vi "CaseStructures.vi"() -> ()   [LabVIEW 2021]
panel:
  in  "Enum":enum16{"Add", "Subtract", "Multiply", "Divide"}(ring)
  in  "stop":bool
  out "Answer":dbl
  in  "Numeber 2":dbl
  in  "Number 1":dbl
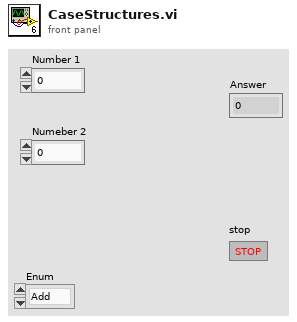
[diagram p1: front panel]
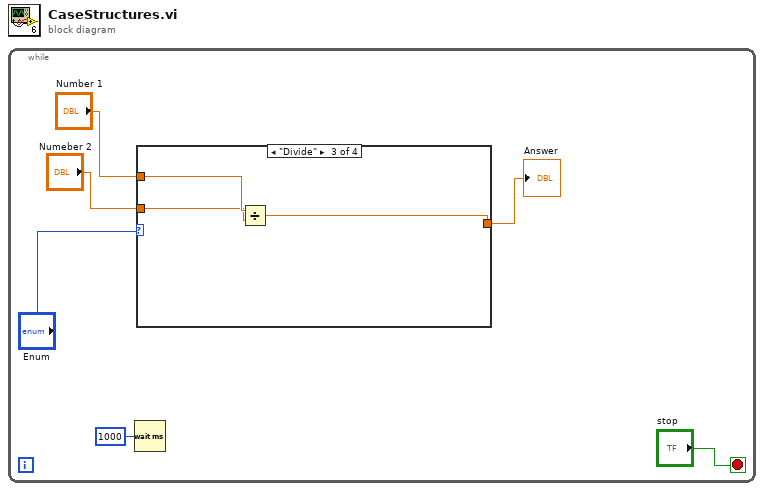
[diagram p0: block diagram]
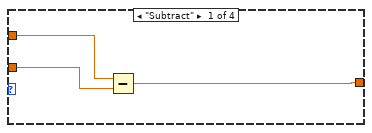
[diagram p2: hidden frame]
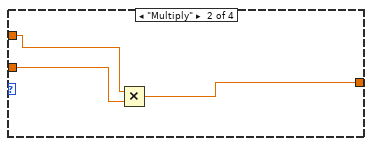
[diagram p3: hidden frame]
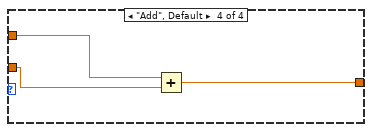
[diagram p4: hidden frame]
diagram:
  n1 = while {
    stop <- "stop" stop-if-true
    n2 = Wait (ms)(milliseconds to wait=u32 1000) -> ()  [unwired: 1 out]
    n3 = case shown="\"Divide\"" "Enum" {
      tunnel: [w7 w10 w13 w18] -> w4
      tunnel: "Number 1" -> [w9 w11 w15 w17]
      tunnel: "Numeber 2" -> [w8 w12 w14 w16]
      frame "Subtract" {
        n4 = Subtract(x=w9, y=w8) -> (x-y=w7:dbl)
      }
      frame "Multiply" {
        n5 = Multiply(x=w11, y=w12) -> (x*y=w10:dbl)
      }
      frame "Divide" {
        n6 = Divide(x=w15, y=w14) -> (x/y=w13:dbl)
      }
      frame "Add", Default {
        n7 = Add(x=w17, y=w16) -> (x+y=w18:dbl)
      }
    }
    "Answer" <- w4
  }
